vi "draw ship.vi"(6 "column":i32, 9 "row":i32, 10 "ship position":u32[][](array[numeric]), 11 "Board in":u32[][](array[numeric])) -> (3 "Board out":u32[][](array[numeric]))   [LabVIEW 2019]
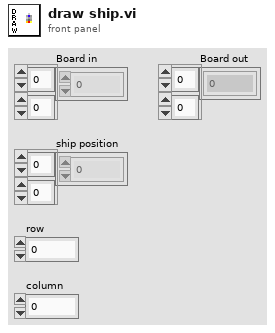
[diagram p1: front panel]
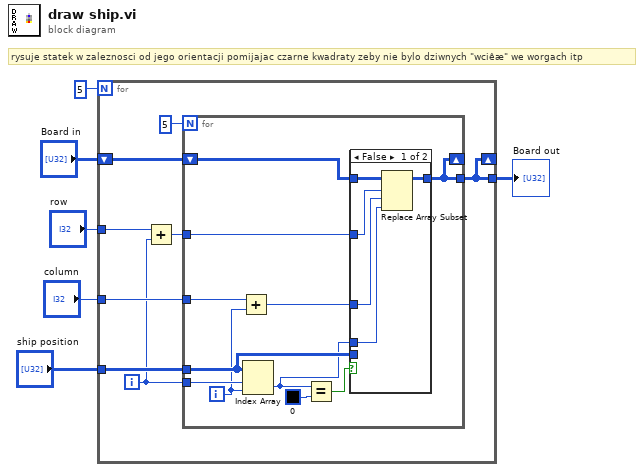
[diagram p0: block diagram]
diagram:
  # "rysuje statek w zaleznosci od jego orientacji pomijajac czarne kwadraty zeby nie bylo dziwnych \"wciêæ\" we worgach itp"
  n1 = for {
    N: 5 -> [_]
    tunnel: "ship position" -> [w14]
    tunnel: "row" -> [w9]
    tunnel: "column" -> [w13]
    shift-right: [w10] -> _
    shift-left: "Board in" -> [w12]
    tunnel: [w10] -> w1
    i -> [w8]
    n2 = Add(x=w9, y=w8) -> (x+y=w7:i32)
    n3 = for {
      N: 5 -> [_]
      tunnel: w14 -> [w22]
      tunnel: w7 -> [w23]
      tunnel: w13 -> [w17]
      shift-right: [w19] -> _
      shift-left: w12 -> [w21]
      tunnel: [w19] -> w10
      tunnel: w8 -> [w18]
      i -> [w15]
      n4 = Add(x=w17, y=w15) -> (x+y=w16:i32)
      n5 = Index Array(array=w22, index (row)=w18, index (col)=w15) -> (element=w20:u32)
      n6 = Equal?(x=w20, y=u32 0 ("Color Box")) -> (x = y?=w24:bool)
      n7 = case shown="False" w24 {
        tunnel: w22 -> [_ _]
        tunnel: w23 -> [w30 _]
        tunnel: w16 -> [w29 _]
        tunnel: w21 -> [w27 w31]
        tunnel: [w26 w31] -> w19
        tunnel: w20 -> [w28 _]
        frame False {
          n8 = Replace Array Subset(array=w27, new element=w28, index (row)=w30, index (col)=w29) -> (w26:u32[][])
        }
        frame True {
        }
      }
    }
  }
  "Board out" <- w1
